vi "Vehicle1.vi"(11 "Interior cargo capacity":dbl=13.1) -> (3 "vehicle":refnum<class "Vehicle.lvclass">)   [LabVIEW 2010]
doc: "Create and initialize a vehicle."
uses:
  Vehicle/Vehicle.lvclass
panel:
  in  "make":string="Company A"
  in  "model":string="car"
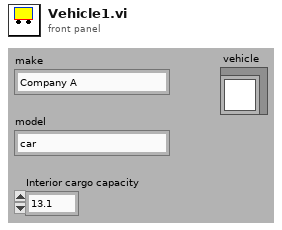
[diagram p1: front panel]
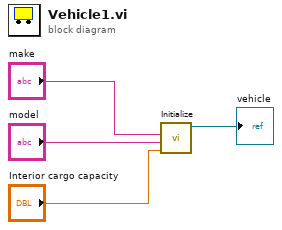
[diagram p0: block diagram]
diagram:
  n1 = call "Initialize.vi"("Interior cargo capacity"="Interior cargo capacity", "model"="model", "make"="make") -> ("vehicle out"=→"vehicle":refnum<class "Vehicle.lvclass">)  [unwired: 8 in]
